vi "UART Read Bytes.vi"(8 "error in (no error)":errorcluster, 10 "UARTIndex":i32, 11 "DevIndex":i32) -> (0 "error out":errorcluster, 1 "function return":i32, 2 "pLen":u16, 3 "pReadData":string)   [LabVIEW 2012, in "ControlUART.lvlib"]
doc: "int WINAPI UART_ReadBytes(int DevIndex,int UARTIndex,unsigned char *pReadData,unsigned short *pLen);"
uses:
  ControlUART.lvlib
  Ginkgo_Driver.dll
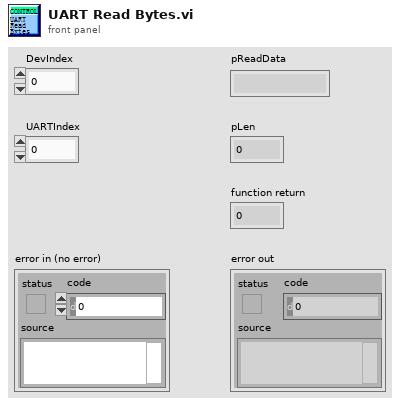
[diagram p1: front panel]
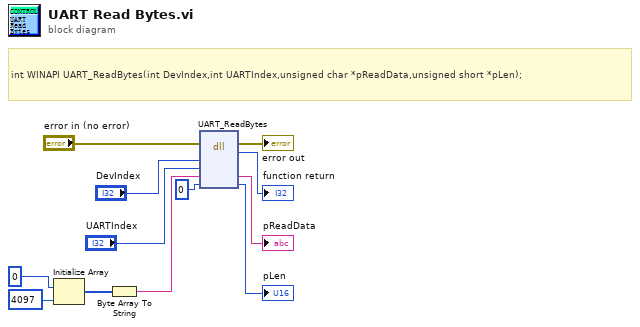
[diagram p0: block diagram]
diagram:
  # "int WINAPI UART_ReadBytes(int DevIndex,int UARTIndex,unsigned char *pReadData,unsigned short *pLen);"
  n1 = Initialize Array(u8 0 ("element"), 4097 ("dimension size")) -> (w9:u8[])
  n2 = Byte Array To String(unsigned byte array=w9) -> (string=w8:string)
  n3 = dll-call lib="E:/Project/vt_ginkgo/truck/Ginkgo Driver/vs2010/Ginkgo_USB-I2C_API_v2.0.3.0/lib/labview_32bit/ControlUART/Ginkgo_Driver.*" fn="UART_ReadBytes"(error in="error in (no error)", "DevIndex"="DevIndex", "UARTIndex"="UARTIndex", "pReadData"=w8, "pLen"=u16 0) -> (error out=→"error out":errorcluster, →"function return":i32, "pReadData"=→"pReadData":string, "pLen"=→"pLen":u16)  [unwired: 4 in, 1 out]
